vi "TraverseStates.vi"(6 "Variant in":variant, 7 "Shift Pressed?":bool, 8 "error in (no error)":errorcluster, 10 "QD Combo Box Ref":refnum<vi>, 11 "QD Launch VI Ref":refnum<vi>) -> (0 "error out":errorcluster, 4 "Variant out":variant)   [LabVIEW 2012]
doc: "Write a 1-2 sentence description of the functionality of your plugin here. Replace the \"$\" below with the character you wish to assign as the default shortcut for this plugin. Do not add any text after the 'Default Shortcut' line below.\n\nDefault Shortcut - [Q]"
panel:
  in  "Undo Name":string="Quick Drop Keyboard Shortcut"
  # "Do not change the connector pane of this VI.\n\nSee the block diagram for directions on how to use this template."
  # "Specify the name of the Undo transaction"
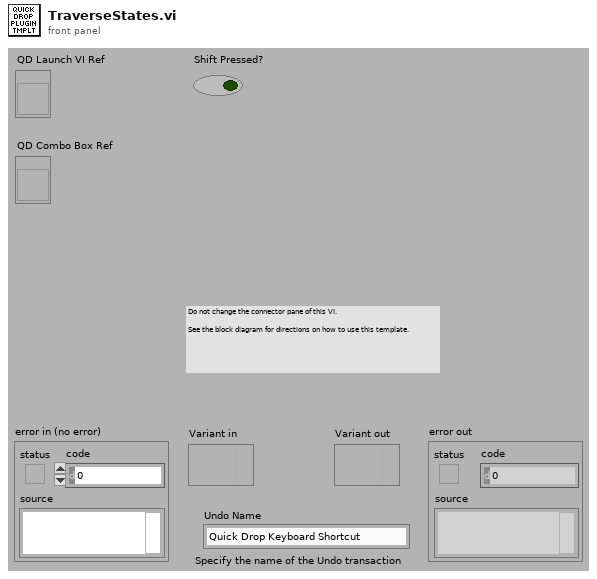
[diagram p1: front panel]
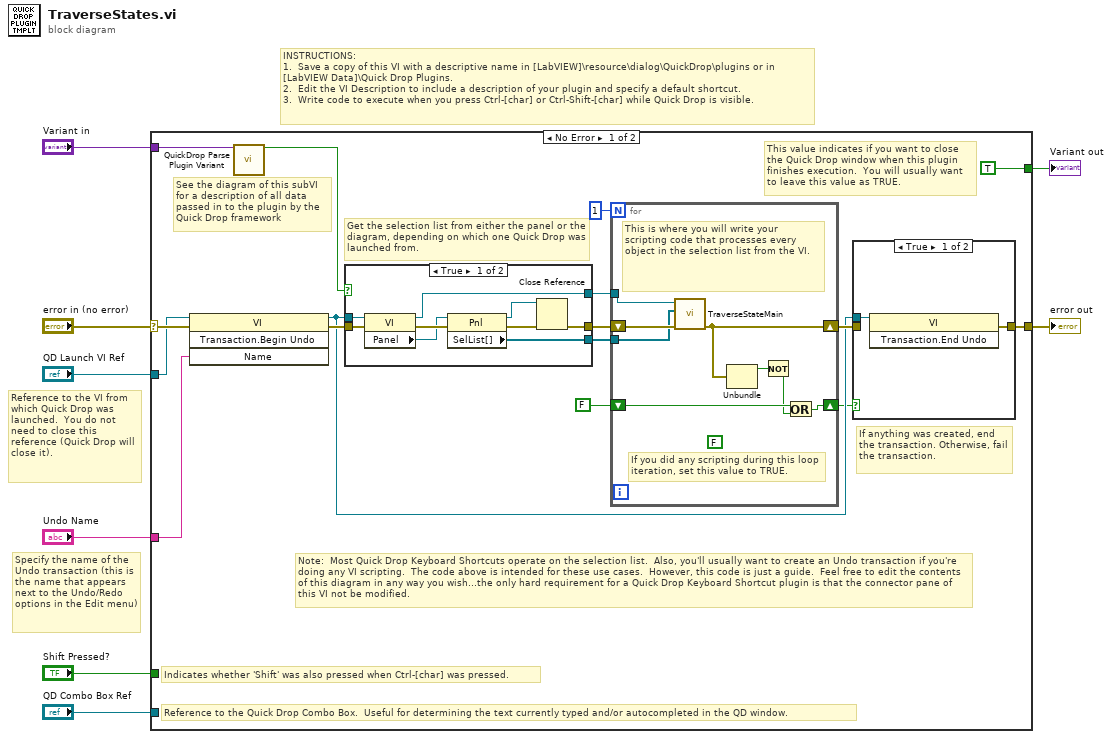
[diagram p0: block diagram]
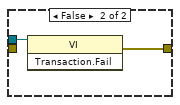
[diagram p2: hidden frame]
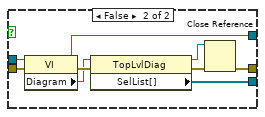
[diagram p3: hidden frame]
diagram:
  # "Specify the name of the Undo transaction (this is the name that appears next to the Undo/Redo options in the Edit menu)"
  # "Reference to the VI from which Quick Drop was launched.  You do not need to close this reference (Quick Drop will close it)."
  # "INSTRUCTIONS:\n1.  Save a copy of this VI with a descriptive name in [LabVIEW]\\resource\\dialog\\QuickDrop\\plugins or in [LabVIEW Data]\\Quick Drop Plugins.\n2.  Edit the VI Description to include a description of your plugin and specify a default shortcut. \n3.  Write code to execute when you press Ctrl-[char] or Ctrl-Shift-[char] while Quick Drop is visible."
  n1 = case shown="No Error" "error in (no error)" {
    selector: "error in (no error)" -> [w23 w55]
    tunnel: [w17 w55] -> w7
    tunnel: "QD Launch VI Ref" -> [w22 _]
    tunnel: "Shift Pressed?" -> [_ _]
    tunnel: "QD Combo Box Ref" -> [_ _]
    tunnel: "Variant in" -> [w24 _]
    tunnel: "Undo Name" -> [w21 _]
    tunnel: [TRUE _] -> w1
    frame No Error {
      # "Note:  Most Quick Drop Keyboard Shortcuts operate on the selection list.  Also, you'll usually want to create an Undo transaction if you're doing any VI scripting.  The code above is intended for these use cases.  However, this code is just a guide.  Feel free to edit the contents of this diagram in any way you wish...the only hard requirement for a Quick Drop Keyboard Shortcut plugin is that the connector pane of this VI not be modified."
      # "Get the selection list from either the panel or the diagram, depending on which one Quick Drop was launched from."
      # "If anything was created, end the transaction. Otherwise, fail the transaction."
      # "This value indicates if you want to close the Quick Drop window when this plugin finishes execution.  You will usually want to leave this value as TRUE."
      # "See the diagram of this subVI for a description of all data passed in to the plugin by the Quick Drop framework"
      # "Reference to the Quick Drop Combo Box.  Useful for determining the text currently typed and/or autocompleted in the QD window."
      # "Indicates whether 'Shift' was also pressed when Ctrl-[char] was pressed."
      n2 = invoke class="VI" method="Transaction.Begin Undo"(reference=w22, error in=w23, "Name"=w21) -> (reference out=w14:refnum<vi>, error out=w18:errorcluster)  [unwired: 1 in, 2 out]
      n3 = call <vilib>:"QuickDrop Parse Plugin Variant.vi"("QDKS Variant in"=w24) -> ("QD Launch VI Panel?"=w19:bool)  [unwired: 12 in, 2 out]
      n4 = case shown="True" w19 {
        tunnel: w18 -> [w45 w54]
        tunnel: w14 -> [w44 w53]
        tunnel: [w39 w48] -> w16
        tunnel: [w38 w47] -> w11
        tunnel: [w37 w46] -> w9
        frame True {
          n5 = property class="VI"(reference=w44, error in=w45) -> (reference out=w37:refnum<vi>, error out=w43:errorcluster, "Panel"=w42:refnum<vi>)
          n6 = property class="Pnl"(reference=w42, error in=w43) -> (reference out=w40:refnum<vi>, error out=w41:errorcluster, "SelList[]"=w38:refnum<vi>[])
          n7 = Close Reference(reference=w40, error in (no error)=w41) -> (error out=w39:errorcluster)
        }
        frame False {
          n8 = property class="VI"(reference=w53, error in=w54) -> (reference out=w46:refnum<vi>, error out=w52:errorcluster, "Diagram"=w51:refnum<vi>)
          n9 = property class="TopLvlDiag"(reference=w51, error in=w52) -> (reference out=w49:refnum<vi>, error out=w50:errorcluster, "SelList[]"=w47:refnum<vi>[])
          n10 = Close Reference(reference=w49, error in (no error)=w50) -> (error out=w48:errorcluster)
        }
      }
      n11 = for {
        N: 1 -> [_]
        shift-right: [w28] -> w15
        shift-left: w16 -> [w30]
        shift-right: [w31] -> w12
        shift-left: FALSE -> [w32]
        tunnel: w11 -> [w25]
        tunnel: w9 -> [w29]
        (unwired) FALSE ("x")
        # "This is where you will write your scripting code that processes every object in the selection list from the VI."
        # "If you did any scripting during this loop iteration, set this value to TRUE."
        n12 = call <resource>:"TraverseStateMain.vi"("error in (no error)"=w30, "SelList[]"=w25, "Vi Ref"=w29) -> ("error out"=w28:errorcluster)  [unwired: 8 in]
        n13 = Unbundle(w28) -> ("status"=w27:bool)  [unwired: 2 out]
        n14 = Not(x=w27) -> (.not. x?=w26:bool)
        n15 = Or(x=w32, y=w26) -> (x .or. y?=w31:bool)
      }
      n16 = case shown="True" w12 {
        tunnel: w14 -> [w33 w35]
        tunnel: [w34 w36] -> w17
        tunnel: w15 -> [_ _]
        frame True {
          n17 = invoke class="VI" method="Transaction.End Undo"(reference=w33) -> (error out=w34:errorcluster)  [unwired: 2 in, 2 out]
        }
        frame False {
          n18 = invoke class="VI" method="Transaction.Fail"(reference=w35) -> (error out=w36:errorcluster)  [unwired: 2 in, 2 out]
        }
      }
    }
    frame Error {
    }
  }
  "error out" <- w7
  "Variant out" <- w1
